vi "CheeseReciveUDP.vi"   [LabVIEW 2013]
uses:
  VisionData.ctl
types:
  T1 = typedef "VisionData.ctl" = cluster{"Total":u8, "Timestamp":u32, "Horizontal":u8, "Vertical":u8, "Left Hot":bool, "Right Hot":bool}
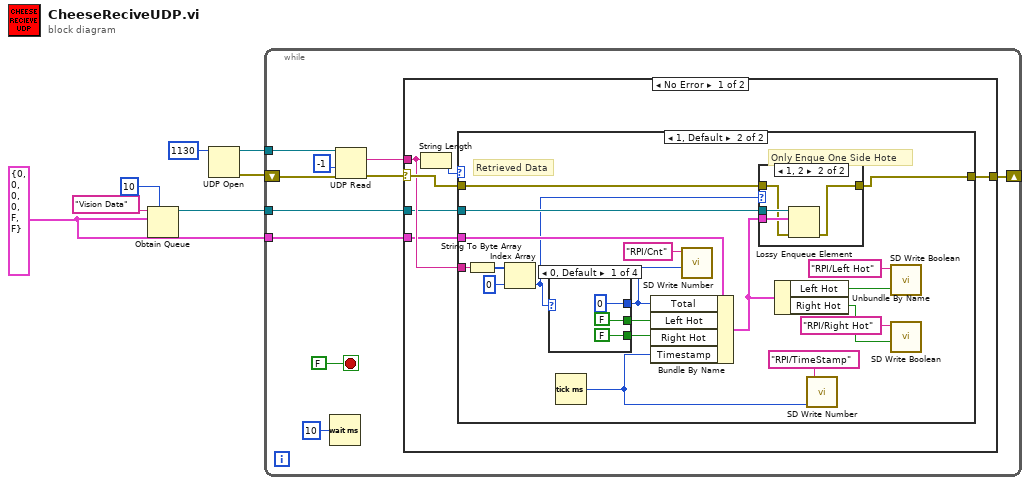
[diagram p0: block diagram]
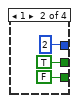
[diagram p4: hidden frame]
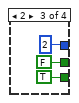
[diagram p5: hidden frame]
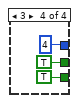
[diagram p6: hidden frame]
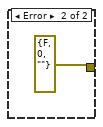
[diagram p7: hidden frame]
diagram:
  w4 = T1 {"Total"=0, "Timestamp"=0, "Horizontal"=0, "Vertical"=0, "Left Hot"=FALSE, "Right Hot"=FALSE}
  n1 = Obtain Queue(max queue size (-1, unlimited)=10, name (unnamed)="Vision Data", element data type=w4) -> (queue out=w5:refnum<queue>)  [unwired: 2 in, 2 out]
  n2 = UDP Open(11:u16 1130 ("port")) -> (port=w1:refnum<k16>, 0:w2:errorcluster)  [unwired: 4 in, 1 out]
  n3 = while {
    shift-right: [w16] -> _
    shift-left: w2 -> [w10]
    tunnel: w5 -> [w15]
    tunnel: w4 -> [w14]
    tunnel: w1 -> [w11]
    stop <- FALSE stop-if-true
    n4 = Wait (ms)(milliseconds to wait=u32 10) -> ()  [unwired: 1 out]
    n5 = UDP Read(connection ID=w11, timeout ms (25000)=-1, 8:w10) -> (data out=w9:string, error out=w8:errorcluster)  [unwired: 1 in, 3 out]
    n6 = case shown="No Error" w8 {
      selector: w8 -> [w22 _]
      tunnel: w9 -> [w20 _]
      tunnel: [w21 errorcluster {"status"=FALSE, "code"=0, "source"=""} ("error IO")] -> w16
      tunnel: w15 -> [w19 _]
      tunnel: w14 -> [w18 _]
      frame No Error {
        n7 = String Length(string=w20) -> (length=w23:i32)
        n8 = case shown="1, Default" w23 {
          tunnel: w22 -> [w24 w27]
          tunnel: [w24 w25] -> w21
          tunnel: w20 -> [_ w36]
          tunnel: w19 -> [_ w33]
          tunnel: w18 -> [_ w32]
          frame 0 {
            # "No Data"
          }
          frame 1, Default {
            # "Only Enque One Side Hote"
            # "Retrieved Data"
            n9 = String To Byte Array(string=w36) -> (unsigned byte array=w35:u8[])
            n10 = Index Array(array=w35, index=0) -> (element=w26:u8)
            n11 = case shown="0, Default" w26 {
              tunnel: [u8 0 ("Total") u8 2 ("Total") u8 2 ("Total") u8 4 ("Total")] -> w29
              tunnel: [FALSE ("Left Hot") TRUE ("Left Hot") FALSE ("Left Hot") TRUE ("Left Hot")] -> w30
              tunnel: [FALSE ("Left Hot") FALSE ("Left Hot") TRUE ("Left Hot") TRUE ("Left Hot")] -> w31
              frame 0, Default {
              }
              frame 1 {
              }
              frame 2 {
              }
              frame 3 {
              }
            }
            n12 = Tick Count (ms)() -> (millisecond timer value=w41:u32)
            n13 = Bundle By Name(cluster=w32, "Total"=w29, "Left Hot"=w30, "Right Hot"=w31, "Timestamp"=w41) -> (w28:T1)
            n14 = call <vilib>:"SD Write Number.vi"("Numeric"=w29, "Name"="RPI/Cnt") -> ()  [unwired: 8 in, 2 out]
            n15 = case shown="1, 2" w26 {
              tunnel: w33 -> [_ w48]
              tunnel: w28 -> [_ w47]
              tunnel: w27 -> [w44 w46]
              tunnel: [w44 w45] -> w25
              frame 0, Default {
              }
              frame 1, 2 {
                n16 = Lossy Enqueue Element(queue=w48, element=w47, error in (no error)=w46) -> (error out=w45:errorcluster)  [unwired: 3 out]
              }
            }
            n17 = Unbundle By Name(w28) -> ("Left Hot"=w40:bool, "Right Hot"=w39:bool)
            n18 = call <vilib>:"SD Write Number.vi"("Numeric"=w41, "Name"="RPI/TimeStamp") -> ()  [unwired: 8 in, 2 out]
            n19 = call <vilib>:"SD Write Boolean.vi"("Boolean"=w40, "Name"="RPI/Left Hot") -> ()  [unwired: 8 in, 2 out]
            n20 = call <vilib>:"SD Write Boolean.vi"("Boolean"=w39, "Name"="RPI/Right Hot") -> ()  [unwired: 8 in, 2 out]
          }
        }
      }
      frame Error {
      }
    }
  }
